vi "test Create Map from Messages to Value Indexes.vi"(8 "error in":errorcluster, 11 "TestCase in":refnum<class "Engine.lvclass">) -> (0 "error out":errorcluster, 3 "TestCase out":refnum<class "Engine.lvclass">)   [LabVIEW 2020, in "Engine.lvclass"]
uses:
  Engine.lvclass
  Shared/1553 Channel.ctl
  Shared/Address.ctl
  Shared/Major Frame Definition.ctl
  Shared/Minor Frame Definition.ctl
  Shared/Message Definition.ctl
  Shared/Message Type.ctl
  Shared/Terminal Endpoint.ctl
  Shared/Parameter Definition.ctl
  Engine/Implementation/Execution Unit/1553 Channel Handles.ctl
  Engine/Implementation/Execution Unit/Message Handles.ctl
  Engine/Implementation/Execution Unit/Parameter Handles.ctl
  <vilib>/NI VeriStand/Custom Device API/Custom Device Item Ref.ctl
  Shared/Error Count Channel Refs.ctl
  Shared/Map of Messages to Value Indexes.ctl
  Shared/Message Map Key.ctl
  Engine/Implementation/Rx Execution Unit/Message Map Value.ctl
  Hardware API/Module Reference.ctl
  <vilib>/addons/_JKI Toolkits/VI Tester/TestCase.llb/TestCase.lvclass
  Engine/Implementation/Rx Execution Unit/Rx Execution Unit.lvclass
  <vilib>/NI VeriStand/Custom Device API/Custom Device API.lvlib
  Engine/Implementation/Execution Unit/Execution Unit.lvclass
  Hardware API/AIM MIL-STD-1553 Hardware API.lvlib
  C:/Program Files (x86)/National Instruments/LabVIEW 2020/vi.lib/addons/_JKI Toolkits/VI Tester/TestCase.llb/TestCase.lvclass
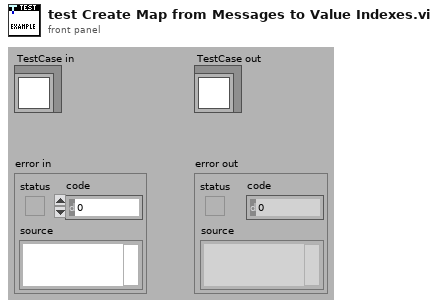
[diagram p1: front panel]
types:
  T1 = typedef "Map of Messages to Value Indexes.ctl" = map{T2, T3}
  T2 = typedef "Message Map Key.ctl" = cluster{"HW channel":u16, "terminal address":u16, "subaddress":u16, "mode code":u16}
  T3 = typedef "AIM MIL-STD-1553 Engine.lvlib/Implementation.lvlib/Rx Execution Unit.lvclass/Message Map Value.ctl" = cluster{"value indexes":i32[], "message":T4, "Tx status count":i32, "Rx status count":i32}
  T4 = typedef "Message Definition.ctl" = cluster{"name":string, "message type":T5, "endpoint Tx":T6, "endpoint Rx":T6, "create timestamp channel":bool, "mode code":u16, "number of words":u16, "parameters":cluster{"name":string, "default value":dbl, "unit":string, "parameter definition":T8}[]}
  T5 = typedef "Message Type.ctl" = string
  T6 = typedef "Terminal Endpoint.ctl" = cluster{"terminal address":T7, "subaddress":T7}
  T7 = typedef "Address.ctl" = u16
  T8 = typedef "Parameter Definition.ctl" = cluster{"start index":i32, "size (bits)":i32, "encoding":enum16{"BNR", "BCD", "Discrete"}, "signed":bool, "multiplier":dbl, "offset":dbl}
  T9 = typedef "AIM MIL-STD-1553 Hardware API.lvlib/Module Reference.ctl" = u32
  T10 = typedef "AIM MIL-STD-1553 Engine.lvlib/Implementation.lvlib/Execution Unit.lvclass/1553 Channel Handles.ctl" = cluster{"messages":T11[], "error count channel refs":T14, "terminal status channels":T13[]}
  T11 = typedef "AIM MIL-STD-1553 Engine.lvlib/Implementation.lvlib/Execution Unit.lvclass/Message Handles.ctl" = cluster{"parameters":T12[], "timestamps":T13[], "Tx status handles":T13[], "Rx status handles":T13[]}
  T12 = typedef "AIM MIL-STD-1553 Engine.lvlib/Implementation.lvlib/Execution Unit.lvclass/Parameter Handles.ctl" = cluster{"Tx channel handle":T13, "RxRT channel handle":T13, "RxBC channel handle":T13}
  T13 = typedef "Custom Device API.lvlib/Custom Device Item Ref.ctl" = u64
  T14 = typedef "Error Count Channel Refs.ctl" = cluster{"general protocol":T13, "improper number of words":T13, "Manchester":T13, "monitor":T13, "parity":T13, "unconfigured frames":T13, "word":T13, "wrong sync":T13}
  T15 = typedef "1553 Channel.ctl" = cluster{"HW channel":u16, "terminal addresses":T7[], "terminal names":string[], "acyclic frame names":string[], "major frames":T16[], "minor frames":T17[], "messages":T4[]}
  T16 = typedef "Major Frame Definition.ctl" = cluster{"name":string, "minor frames":string[]}
  T17 = typedef "Minor Frame Definition.ctl" = cluster{"name":string, "messages":string[]}
  T18 = typedef "AIM MIL-STD-1553 Engine.lvlib/Implementation.lvlib/Rx Execution Unit.lvclass/Status Terminal Lookup Data.ctl" = cluster{"value index":i32, "remote terminal handle":u64, "terminal address":u64}
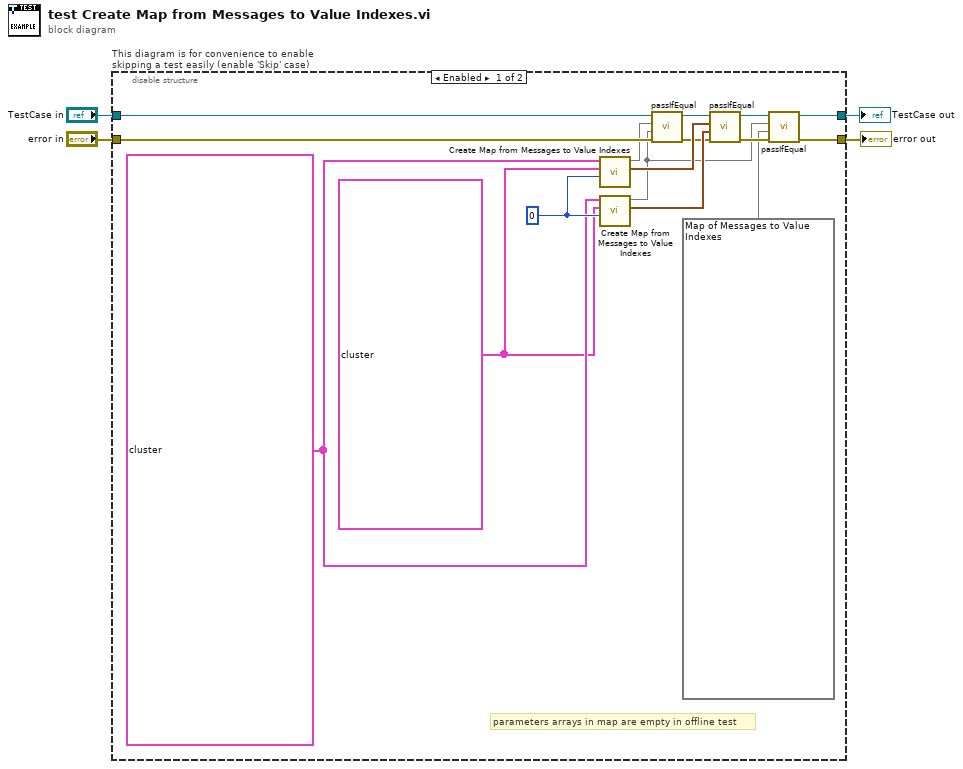
[diagram p0: block diagram]
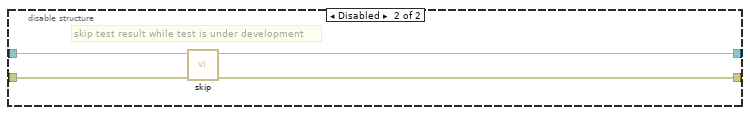
[diagram p2: hidden frame]
diagram:
  n1 = disable-structure "This diagram is for convenience to enable skipping a test easily (enable 'Skip' case)" shown="Enabled" {
    disable-tunnel: "TestCase in" -> [w14 w24]
    disable-tunnel: [w20 w22] -> w1
    disable-tunnel: [w19 w23] -> w3
    disable-tunnel: "error in" -> [w15 w21]
    frame Enabled {
      w18 = T9 0 ("module reference")
      w16 = T10[] [{"messages"=[{"parameters"=[{"Tx channel handle"=18446744073709551615, "RxRT channel handle"=18446744073709551615, "RxBC channel handle"=0}, {"Tx channel handle"=18446744073709551615, "RxRT channel handle"=18446744073709551615, "RxBC channel handle"=0}, {"Tx channel handle"=18446744073709551615, "RxRT channel handle"=18446744073709551615, "RxBC channel handle"=0}], "timestamps"=[], "Tx status handles"=[], "Rx status handles"=[]}, {"parameters"=[{"Tx channel handle"=18446744073709551615, "RxRT channel handle"=18446744073709551615, "RxBC channel handle"=18446744073709551615}, {"Tx channel handle"=18446744073709551615, "RxRT channel handle"=18446744073709551615, "RxBC channel handle"=18446744073709551615}, {"Tx channel handle"=18446744073709551615, "RxRT channel handle"=18446744073709551615, "RxBC channel handle"=18446744073709551615}, {"Tx channel handle"=18446744073709551615, "RxRT channel handle"=18446744073709551615, "RxBC channel handle"=18446744073709551615}, {"Tx channel handle"=18446744073709551615, "RxRT channel handle"=18446744073709551615, "RxBC channel handle"=18446744073709551615}, {"Tx channel handle"=18446744073709551615, "RxRT channel handle"=18446744073709551615, "RxBC channel handle"=18446744073709551615}, {"Tx channel handle"=18446744073709551615, "RxRT channel handle"=18446744073709551615, "RxBC channel handle"=18446744073709551615}, {"Tx channel handle"=18446744073709551615, "RxRT channel handle"=18446744073709551615, "RxBC channel handle"=18446744073709551615}, {"Tx channel handle"=18446744073709551615, "RxRT channel handle"=18446744073709551615, "RxBC channel handle"=18446744073709551615}, {"Tx channel handle"=18446744073709551615, "RxRT channel handle"=18446744073709551615, "RxBC channel handle"=18446744073709551615}, {"Tx channel handle"=18446744073709551615, "RxRT channel handle"=18446744073709551615, "RxBC channel handle"=18446744073709551615}], "timestamps"=[], "Tx status handles"=[], "Rx status handles"=[]}, {"parameters"=[{"Tx channel handle"=18446744073709551615, "RxRT channel handle"=18446744073709551615, "RxBC channel handle"=0}, {"Tx channel handle"=18446744073709551615, "RxRT channel handle"=18446744073709551615, "RxBC channel handle"=0}, {"Tx channel handle"=18446744073709551615, "RxRT channel handle"=18446744073709551615, "RxBC channel handle"=0}, {"Tx channel handle"=18446744073709551615, "RxRT channel handle"=18446744073709551615, "RxBC channel handle"=0}], "timestamps"=[], "Tx status handles"=[], "Rx status handles"=[]}, {"parameters"=[{"Tx channel handle"=18446744073709551615, "RxRT channel handle"=0, "RxBC channel handle"=18446744073709551615}, {"Tx channel handle"=18446744073709551615, "RxRT channel handle"=0, "RxBC channel handle"=18446744073709551615}, {"Tx channel handle"=18446744073709551615, "RxRT channel handle"=0, "RxBC channel handle"=18446744073709551615}, {"Tx channel handle"=18446744073709551615, "RxRT channel handle"=0, "RxBC channel handle"=18446744073709551615}, {"Tx channel handle"=18446744073709551615, "RxRT channel handle"=0, "RxBC channel handle"=18446744073709551615}, {"Tx channel handle"=18446744073709551615, "RxRT channel handle"=0, "RxBC channel handle"=18446744073709551615}], "timestamps"=[], "Tx status handles"=[], "Rx status handles"=[]}, {"parameters"=[{"Tx channel handle"=18446744073709551615, "RxRT channel handle"=0, "RxBC channel handle"=18446744073709551615}, {"Tx channel handle"=18446744073709551615, "RxRT channel handle"=0, "RxBC channel handle"=18446744073709551615}], "timestamps"=[], "Tx status handles"=[], "Rx status handles"=[]}, {"parameters"=[{"Tx channel handle"=18446744073709551615, "RxRT channel handle"=18446744073709551615, "RxBC channel handle"=18446744073709551615}, {"Tx channel handle"=18446744073709551615, "RxRT channel handle"=18446744073709551615, "RxBC channel handle"=18446744073709551615}, {"Tx channel handle"=18446744073709551615, "RxRT channel handle"=18446744073709551615, "RxBC channel handle"=18446744073709551615}, {"Tx channel handle"=18446744073709551615, "RxRT channel handle"=18446744073709551615, "RxBC channel handle"=18446744073709551615}], "timestamps"=[], "Tx status handles"=[], "Rx status handles"=[]}, {"parameters"=[{"Tx channel handle"=18446744073709551615, "RxRT channel handle"=0, "RxBC channel handle"=18446744073709551615}], "timestamps"=[], "Tx status handles"=[], "Rx status handles"=[]}, {"parameters"=[{"Tx channel handle"=18446744073709551615, "RxRT channel handle"=18446744073709551615, "RxBC channel handle"=0}], "timestamps"=[], "Tx status handles"=[], "Rx status handles"=[]}, {"parameters"=[{"Tx channel handle"=18446744073709551615, "RxRT channel handle"=18446744073709551615, "RxBC channel handle"=0}, {"Tx channel handle"=18446744073709551615, "RxRT channel handle"=18446744073709551615, "RxBC channel handle"=0}, {"Tx channel handle"=18446744073709551615, "RxRT channel handle"=18446744073709551615, "RxBC channel handle"=0}, {"Tx channel handle"=18446744073709551615, "RxRT channel handle"=18446744073709551615, "RxBC channel handle"=0}, {"Tx channel handle"=18446744073709551615, "RxRT channel handle"=18446744073709551615, "RxBC channel handle"=0}, {"Tx channel handle"=18446744073709551615, "RxRT channel handle"=18446744073709551615, "RxBC channel handle"=0}], "timestamps"=[], "Tx status handles"=[], "Rx status handles"=[]}], "error count channel refs"={"general protocol"=18446744073709551615, "improper number of words"=18446744073709551615, "Manchester"=18446744073709551615, "monitor"=18446744073709551615, "parity"=18446744073709551615, "unconfigured frames"=18446744073709551615, "word"=18446744073709551615, "wrong sync"=18446744073709551615}, "terminal status channels"=[]}] ("1553 channel handles")
      w17 = T15[] [{"HW channel"=0, "terminal addresses"=[], "terminal names"=[], "acyclic frame names"=[], "major frames"=[], "minor frames"=[], "messages"=[{"name"="BC 2 RT 1", "message type"="BC to RT", "endpoint Tx"={"terminal address"=0, "subaddress"=0}, "endpoint Rx"={"terminal address"=1, "subaddress"=2}, "create timestamp channel"=FALSE, "mode code"=0, "number of words"=3, "parameters"=[{"name"="", "default value"=1.0, "unit"="", "parameter definition"={"start index"=0, "size (bits)"=16, "encoding"=enum."BNR", "signed"=FALSE, "multiplier"=1.0, "offset"=0.0}}, {"name"="", "default value"=1.0, "unit"="", "parameter definition"={"start index"=16, "size (bits)"=16, "encoding"=enum."BNR", "signed"=FALSE, "multiplier"=1.0, "offset"=0.0}}, {"name"="", "default value"=1.0, "unit"="", "parameter definition"={"start index"=32, "size (bits)"=16, "encoding"=enum."BNR", "signed"=FALSE, "multiplier"=1.0, "offset"=0.0}}]}, {"name"="RT 2 RT 2", "message type"="RT to RT", "endpoint Tx"={"terminal address"=15, "subaddress"=21}, "endpoint Rx"={"terminal address"=31, "subaddress"=21}, "create timestamp channel"=FALSE, "mode code"=0, "number of words"=11, "parameters"=[{"name"="", "default value"=1.0, "unit"="", "parameter definition"={"start index"=0, "size (bits)"=16, "encoding"=enum."BNR", "signed"=FALSE, "multiplier"=2.0, "offset"=0.0}}, {"name"="", "default value"=1.0, "unit"="", "parameter definition"={"start index"=16, "size (bits)"=16, "encoding"=enum."BNR", "signed"=FALSE, "multiplier"=1.0, "offset"=50.0}}, {"name"="", "default value"=1.0, "unit"="", "parameter definition"={"start index"=32, "size (bits)"=16, "encoding"=enum."BNR", "signed"=TRUE, "multiplier"=1.0, "offset"=0.0}}, {"name"="", "default value"=1.0, "unit"="", "parameter definition"={"start index"=48, "size (bits)"=16, "encoding"=enum."BNR", "signed"=FALSE, "multiplier"=1.0, "offset"=0.0}}, {"name"="", "default value"=1.0, "unit"="", "parameter definition"={"start index"=64, "size (bits)"=16, "encoding"=enum."BNR", "signed"=FALSE, "multiplier"=1.0, "offset"=0.0}}, {"name"="", "default value"=1.0, "unit"="", "parameter definition"={"start index"=80, "size (bits)"=16, "encoding"=enum."BNR", "signed"=FALSE, "multiplier"=1.0, "offset"=0.0}}, {"name"="", "default value"=1.0, "unit"="", "parameter definition"={"start index"=96, "size (bits)"=16, "encoding"=enum."BNR", "signed"=FALSE, "multiplier"=1.0, "offset"=0.0}}, {"name"="", "default value"=1.0, "unit"="", "parameter definition"={"start index"=112, "size (bits)"=16, "encoding"=enum."BNR", "signed"=FALSE, "multiplier"=1.0, "offset"=0.0}}, {"name"="", "default value"=1.0, "unit"="", "parameter definition"={"start index"=128, "size (bits)"=16, "encoding"=enum."BNR", "signed"=FALSE, "multiplier"=1.0, "offset"=0.0}}, {"name"="", "default value"=1.0, "unit"="", "parameter definition"={"start index"=144, "size (bits)"=16, "encoding"=enum."BNR", "signed"=FALSE, "multiplier"=1.0, "offset"=0.0}}, {"name"="", "default value"=1.0, "unit"="", "parameter definition"={"start index"=160, "size (bits)"=16, "encoding"=enum."BNR", "signed"=FALSE, "multiplier"=1.0, "offset"=0.0}}]}, {"name"="BC 2 RT 2", "message type"="BC to RT", "endpoint Tx"={"terminal address"=0, "subaddress"=0}, "endpoint Rx"={"terminal address"=1, "subaddress"=3}, "create timestamp channel"=FALSE, "mode code"=0, "number of words"=4, "parameters"=[{"name"="", "default value"=1.0, "unit"="", "parameter definition"={"start index"=0, "size (bits)"=16, "encoding"=enum."BNR", "signed"=FALSE, "multiplier"=1.0, "offset"=0.0}}, {"name"="", "default value"=1.0, "unit"="", "parameter definition"={"start index"=16, "size (bits)"=16, "encoding"=enum."BNR", "signed"=FALSE, "multiplier"=1.0, "offset"=0.0}}, {"name"="", "default value"=1.0, "unit"="", "parameter definition"={"start index"=32, "size (bits)"=16, "encoding"=enum."BNR", "signed"=FALSE, "multiplier"=1.0, "offset"=0.0}}, {"name"="", "default value"=1.0, "unit"="", "parameter definition"={"start index"=48, "size (bits)"=16, "encoding"=enum."BNR", "signed"=FALSE, "multiplier"=1.0, "offset"=0.0}}]}, {"name"="RT 2 BC 1", "message type"="RT to BC", "endpoint Tx"={"terminal address"=1, "subaddress"=5}, "endpoint Rx"={"terminal address"=0, "subaddress"=0}, "create timestamp channel"=FALSE, "mode code"=0, "number of words"=6, "parameters"=[{"name"="", "default value"=1.0, "unit"="", "parameter definition"={"start index"=0, "size (bits)"=16, "encoding"=enum."BNR", "signed"=FALSE, "multiplier"=1.0, "offset"=0.0}}, {"name"="", "default value"=1.0, "unit"="", "parameter definition"={"start index"=16, "size (bits)"=16, "encoding"=enum."BNR", "signed"=FALSE, "multiplier"=1.0, "offset"=0.0}}, {"name"="", "default value"=1.0, "unit"="", "parameter definition"={"start index"=32, "size (bits)"=16, "encoding"=enum."BNR", "signed"=FALSE, "multiplier"=1.0, "offset"=0.0}}, {"name"="", "default value"=1.0, "unit"="", "parameter definition"={"start index"=48, "size (bits)"=16, "encoding"=enum."BNR", "signed"=FALSE, "multiplier"=1.0, "offset"=0.0}}, {"name"="", "default value"=1.0, "unit"="", "parameter definition"={"start index"=64, "size (bits)"=16, "encoding"=enum."BNR", "signed"=FALSE, "multiplier"=1.0, "offset"=0.0}}, {"name"="", "default value"=1.0, "unit"="", "parameter definition"={"start index"=80, "size (bits)"=16, "encoding"=enum."BNR", "signed"=FALSE, "multiplier"=1.0, "offset"=0.0}}]}, {"name"="RT 2 BC 2", "message type"="RT to BC", "endpoint Tx"={"terminal address"=1, "subaddress"=6}, "endpoint Rx"={"terminal address"=0, "subaddress"=0}, "create timestamp channel"=FALSE, "mode code"=0, "number of words"=2, "parameters"=[{"name"="", "default value"=1.0, "unit"="", "parameter definition"={"start index"=0, "size (bits)"=16, "encoding"=enum."BNR", "signed"=FALSE, "multiplier"=1.0, "offset"=0.0}}, {"name"="", "default value"=1.0, "unit"="", "parameter definition"={"start index"=16, "size (bits)"=16, "encoding"=enum."BNR", "signed"=FALSE, "multiplier"=1.0, "offset"=0.0}}]}, {"name"="RT 2 RT 1", "message type"="RT to RT", "endpoint Tx"={"terminal address"=1, "subaddress"=20}, "endpoint Rx"={"terminal address"=15, "subaddress"=20}, "create timestamp channel"=FALSE, "mode code"=0, "number of words"=4, "parameters"=[{"name"="", "default value"=1.0, "unit"="", "parameter definition"={"start index"=0, "size (bits)"=16, "encoding"=enum."BNR", "signed"=FALSE, "multiplier"=1.0, "offset"=0.0}}, {"name"="", "default value"=1.0, "unit"="", "parameter definition"={"start index"=16, "size (bits)"=16, "encoding"=enum."BNR", "signed"=FALSE, "multiplier"=1.0, "offset"=0.0}}, {"name"="", "default value"=1.0, "unit"="", "parameter definition"={"start index"=32, "size (bits)"=16, "encoding"=enum."BNR", "signed"=FALSE, "multiplier"=1.0, "offset"=0.0}}, {"name"="", "default value"=1.0, "unit"="", "parameter definition"={"start index"=48, "size (bits)"=16, "encoding"=enum."BNR", "signed"=FALSE, "multiplier"=1.0, "offset"=0.0}}]}, {"name"="MC 16", "message type"="MC", "endpoint Tx"={"terminal address"=1, "subaddress"=31}, "endpoint Rx"={"terminal address"=0, "subaddress"=0}, "create timestamp channel"=FALSE, "mode code"=16, "number of words"=0, "parameters"=[{"name"="", "default value"=1.0, "unit"="", "parameter definition"={"start index"=0, "size (bits)"=16, "encoding"=enum."BNR", "signed"=FALSE, "multiplier"=1.0, "offset"=0.0}}]}, {"name"="MC 17", "message type"="MC", "endpoint Tx"={"terminal address"=0, "subaddress"=0}, "endpoint Rx"={"terminal address"=1, "subaddress"=31}, "create timestamp channel"=FALSE, "mode code"=17, "number of words"=0, "parameters"=[{"name"="", "default value"=1.0, "unit"="", "parameter definition"={"start index"=0, "size (bits)"=16, "encoding"=enum."BNR", "signed"=FALSE, "multiplier"=1.0, "offset"=0.0}}]}, {"name"="BC 2 RT 4", "message type"="BC to RT", "endpoint Tx"={"terminal address"=0, "subaddress"=0}, "endpoint Rx"={"terminal address"=31, "subaddress"=28}, "create timestamp channel"=FALSE, "mode code"=0, "number of words"=6, "parameters"=[{"name"="", "default value"=1.0, "unit"="", "parameter definition"={"start index"=0, "size (bits)"=16, "encoding"=enum."BNR", "signed"=FALSE, "multiplier"=1.0, "offset"=0.0}}, {"name"="", "default value"=1.0, "unit"="", "parameter definition"={"start index"=16, "size (bits)"=16, "encoding"=enum."BNR", "signed"=FALSE, "multiplier"=1.0, "offset"=0.0}}, {"name"="", "default value"=1.0, "unit"="", "parameter definition"={"start index"=32, "size (bits)"=16, "encoding"=enum."BNR", "signed"=FALSE, "multiplier"=1.0, "offset"=0.0}}, {"name"="", "default value"=1.0, "unit"="", "parameter definition"={"start index"=48, "size (bits)"=16, "encoding"=enum."BNR", "signed"=FALSE, "multiplier"=1.0, "offset"=0.0}}, {"name"="", "default value"=1.0, "unit"="", "parameter definition"={"start index"=64, "size (bits)"=16, "encoding"=enum."BNR", "signed"=FALSE, "multiplier"=1.0, "offset"=0.0}}, {"name"="", "default value"=1.0, "unit"="", "parameter definition"={"start index"=80, "size (bits)"=16, "encoding"=enum."BNR", "signed"=FALSE, "multiplier"=1.0, "offset"=0.0}}]}, {"name"="MC 1", "message type"="MC", "endpoint Tx"={"terminal address"=0, "subaddress"=0}, "endpoint Rx"={"terminal address"=31, "subaddress"=31}, "create timestamp channel"=FALSE, "mode code"=1, "number of words"=0, "parameters"=[]}]}] ("1553 channels")
      # "parameters arrays in map are empty in offline test"
      n2 = call "Create Map from Messages to Value Indexes.vi"("module reference"=w18, "1553 channel handles"=w16, "1553 channels"=w17) -> ("status lookup data"=w12:T18[], "map from messages to value indexes"=w13:T1)  [unwired: 5 in, 2 out]
      n3 = call "Create Map from Messages to Value Indexes.vi"("module reference"=w18, "1553 channel handles"=w16, "1553 channels"=w17) -> ("status lookup data"=w11:T18[], "map from messages to value indexes"=w6:T1)  [unwired: 5 in, 2 out]
      n4 = call-dynamic "passIfEqual.vi"("error in (no error)"=w15, "y"=w6, "x"=w13, "TestCase in"=w14) -> ("error out"=w9:errorcluster, "TestCase out"=w10:refnum<class "Engine.lvclass">)  [unwired: 6 in]
      n5 = call-dynamic "passIfEqual.vi"("error in (no error)"=w9, "y"=w11, "x"=w12, "TestCase in"=w10) -> ("error out"=w7:errorcluster, "TestCase out"=w8:refnum<class "Engine.lvclass">)  [unwired: 6 in]
      n6 = call-dynamic "passIfEqual.vi"("error in (no error)"=w7, "y"=T1 {{"HW channel"=0, "terminal address"=1, "subaddress"=2, "mode code"=0}={"value indexes"=[], "message"={"name"="BC 2 RT 1", "message type"="BC to RT", "endpoint Tx"={"terminal address"=0, "subaddress"=0}, "endpoint Rx"={"terminal address"=1, "subaddress"=2}, "create timestamp channel"=FALSE, "mode code"=0, "number of words"=3, "parameters"=[]}, "Tx status count"=0, "Rx status count"=0}, {"HW channel"=0, "terminal address"=1, "subaddress"=3, "mode code"=0}={"value indexes"=[], "message"={"name"="BC 2 RT 2", "message type"="BC to RT", "endpoint Tx"={"terminal address"=0, "subaddress"=0}, "endpoint Rx"={"terminal address"=1, "subaddress"=3}, "create timestamp channel"=FALSE, "mode code"=0, "number of words"=4, "parameters"=[]}, "Tx status count"=0, "Rx status count"=0}, {"HW channel"=0, "terminal address"=1, "subaddress"=5, "mode code"=0}={"value indexes"=[], "message"={"name"="RT 2 BC 1", "message type"="RT to BC", "endpoint Tx"={"terminal address"=1, "subaddress"=5}, "endpoint Rx"={"terminal address"=0, "subaddress"=0}, "create timestamp channel"=FALSE, "mode code"=0, "number of words"=6, "parameters"=[]}, "Tx status count"=0, "Rx status count"=0}, {"HW channel"=0, "terminal address"=1, "subaddress"=6, "mode code"=0}={"value indexes"=[], "message"={"name"="RT 2 BC 2", "message type"="RT to BC", "endpoint Tx"={"terminal address"=1, "subaddress"=6}, "endpoint Rx"={"terminal address"=0, "subaddress"=0}, "create timestamp channel"=FALSE, "mode code"=0, "number of words"=2, "parameters"=[]}, "Tx status count"=0, "Rx status count"=0}, {"HW channel"=0, "terminal address"=1, "subaddress"=31, "mode code"=16}={"value indexes"=[], "message"={"name"="MC 16", "message type"="MC", "endpoint Tx"={"terminal address"=1, "subaddress"=31}, "endpoint Rx"={"terminal address"=0, "subaddress"=0}, "create timestamp channel"=FALSE, "mode code"=16, "number of words"=0, "parameters"=[]}, "Tx status count"=0, "Rx status count"=0}, {"HW channel"=0, "terminal address"=1, "subaddress"=31, "mode code"=17}={"value indexes"=[], "message"={"name"="MC 17", "message type"="MC", "endpoint Tx"={"terminal address"=0, "subaddress"=0}, "endpoint Rx"={"terminal address"=1, "subaddress"=31}, "create timestamp channel"=FALSE, "mode code"=17, "number of words"=0, "parameters"=[]}, "Tx status count"=0, "Rx status count"=0}, {"HW channel"=0, "terminal address"=15, "subaddress"=20, "mode code"=0}={"value indexes"=[], "message"={"name"="RT 2 RT 1", "message type"="RT to RT", "endpoint Tx"={"terminal address"=1, "subaddress"=20}, "endpoint Rx"={"terminal address"=15, "subaddress"=20}, "create timestamp channel"=FALSE, "mode code"=0, "number of words"=4, "parameters"=[]}, "Tx status count"=0, "Rx status count"=0}, {"HW channel"=0, "terminal address"=31, "subaddress"=21, "mode code"=0}={"value indexes"=[], "message"={"name"="RT 2 RT 2", "message type"="RT to RT", "endpoint Tx"={"terminal address"=15, "subaddress"=21}, "endpoint Rx"={"terminal address"=31, "subaddress"=21}, "create timestamp channel"=FALSE, "mode code"=0, "number of words"=11, "parameters"=[]}, "Tx status count"=0, "Rx status count"=0}, {"HW channel"=0, "terminal address"=31, "subaddress"=28, "mode code"=0}={"value indexes"=[], "message"={"name"="BC 2 RT 4", "message type"="BC to RT", "endpoint Tx"={"terminal address"=0, "subaddress"=0}, "endpoint Rx"={"terminal address"=31, "subaddress"=28}, "create timestamp channel"=FALSE, "mode code"=0, "number of words"=6, "parameters"=[]}, "Tx status count"=0, "Rx status count"=0}} ("map from messages to value indexes"), "x"=w6, "TestCase in"=w8) -> ("error out"=w19:errorcluster, "TestCase out"=w20:refnum<class "Engine.lvclass">)  [unwired: 6 in]
    }
    frame Disabled {
      # "skip test result while test is under development"
      n7 = call <vilib>:"skip.vi"("error in (no error)"=w21, "TestCase in"=w24) -> ("error out"=w23:errorcluster, "TestCase out"=w22:refnum<class "Engine.lvclass">)  [unwired: 8 in]
    }
  }
  "error out" <- w3
  "TestCase out" <- w1
